vi "Convert 1DWfm to DDT.vi"(2 "Array of Waveforms":waveform(dbl)[](array[waveform])) -> (4 "Dynamic Data Type":dynamicdata(graph))   [LabVIEW 2020]
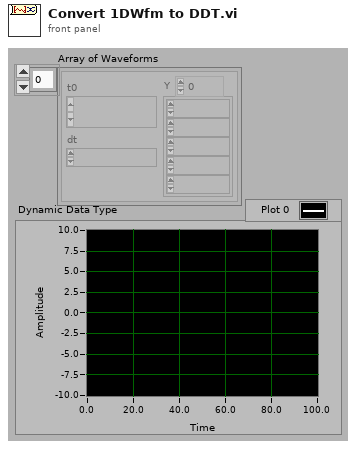
[diagram p1: front panel]
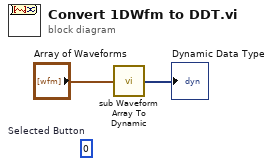
[diagram p0: block diagram]
diagram:
  (unwired) u32 0  # Selected Button
  n1 = call "sub Waveform Array To Dynamic.vi"("Input"="Array of Waveforms") -> ("Output"=→"Dynamic Data Type":dynamicdata)  [unwired: 4 out]
